vi "GetVIByName.vi"(0 "Application Ref in":refnum<vi>, 5 "VI Name":string, 11 "error in (no error)":errorcluster) -> (4 "Application Ref out":refnum<vi>, 6 "VI Reference":refnum<vi>, 15 "error out":errorcluster)   [LabVIEW 2016]
doc: "Gives the reference of the specified VI in the input"
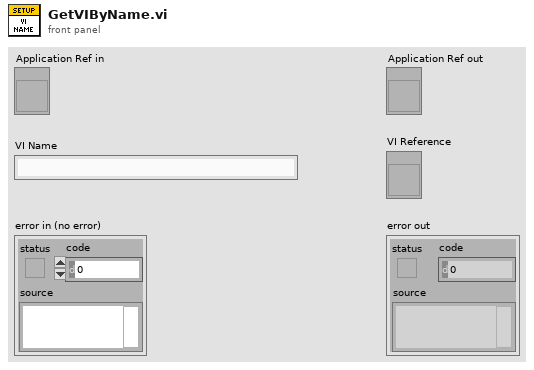
[diagram p1: front panel]
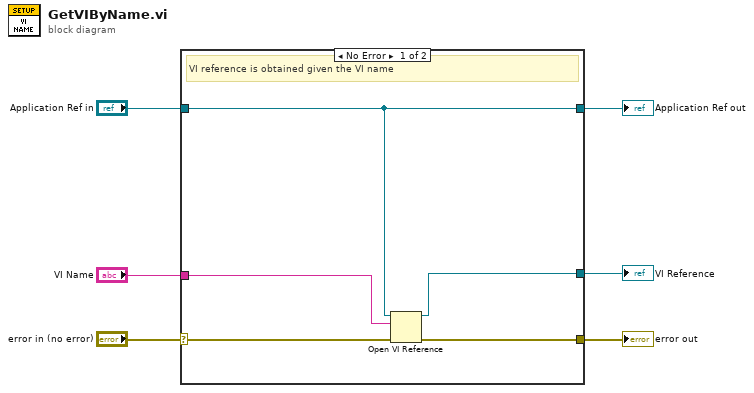
[diagram p0: block diagram]
diagram:
  n1 = case shown="No Error" "error in (no error)" {
    selector: "error in (no error)" -> [w11 w13]
    tunnel: [w10 w13] -> w5
    tunnel: [w9 w12] -> w3
    tunnel: "Application Ref in" -> [w9 w12]
    tunnel: "VI Name" -> [w8 _]
    tunnel: [w7 _] -> w1
    frame No Error {
      # "VI reference is obtained given the VI name"
      n2 = Open VI Reference(application reference (local)=w9, vi path=w8, error in (no error)=w11) -> (vi reference=w7:refnum<vi>, error out=w10:errorcluster)  [unwired: 3 in]
    }
    frame Error {
    }
  }
  "error out" <- w5
  "Application Ref out" <- w3
  "VI Reference" <- w1
